vi "(SubVI) Change ADC and DAC Rate of Stage_YCC.vi"(0 "ADC Rate for 20bit (ms)":T2(ring)=enum."3750 Hz", 2 "Tab Control":T1(tab), 3 "DAC rate (ms)":dbl=5.0) -> (5 "Sampling Rate for reading (Hz)":dbl, 6 "DAC rate (Hz)":dbl)   [LabVIEW 2014]
uses:
  Main-Stage-PI/(Global) Current handle and LaserPower_YCC.vi
  MCL-dll-Labview 32-bit/Madlib.dll
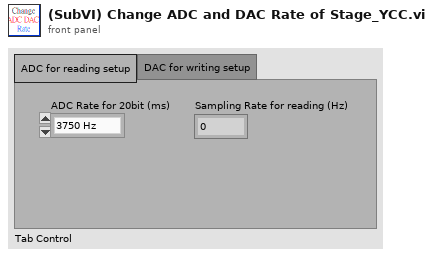
[diagram p1: front panel]
types:
  T1 = enum32{"ADC for reading setup", "DAC for writing setup"}
  T2 = enum16{"50 Hz", "60 Hz", "100 Hz", "500 Hz", "1000 Hz", "2000 Hz", "3750 Hz"}
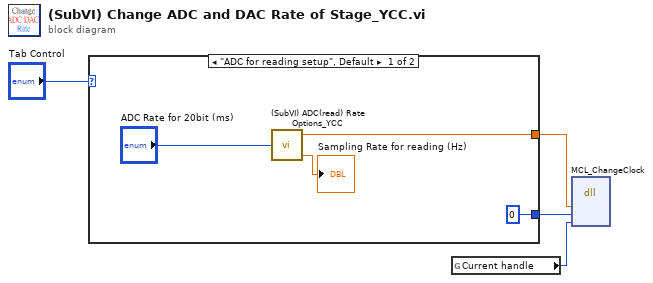
[diagram p0: block diagram]
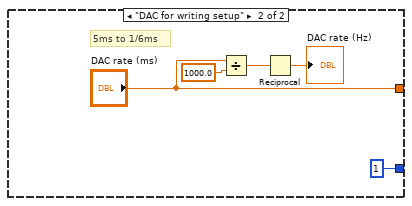
[diagram p2: hidden frame]
diagram:
  n1 = case shown="\"ADC for reading setup\", Default" "Tab Control" {
    tunnel: [0 1] -> w3
    tunnel: [w6 "DAC rate (ms)"] -> w1
    frame "ADC for reading setup", Default {
      n2 = call "(SubVI) ADC(read) Rate Options_YCC.vi"("ADC Rate for 20bit (ms)"="ADC Rate for 20bit (ms)") -> ("Sampling Rate for reading (Hz)"=→"Sampling Rate for reading (Hz)":dbl, "waiting code for Reading (20bits)"=w6:dbl)  [unwired: 3 in]
    }
    frame "DAC for writing setup" {
      # "5ms to 1/6ms"
      n3 = Divide(x="DAC rate (ms)", y=1000.0) -> (x/y=w12:dbl)
      n4 = Reciprocal(x=w12) -> (1/x=→"DAC rate (Hz)":dbl)
    }
  }
  n5 = global read "(Global) Current handle and LaserPower_YCC.vi" "Current handle"() -> (w4:i32)
  n6 = dll-call lib="C:/Users/hwlab/OneDrive - g.ntu.edu.tw/OT/YCC's OT-PI/Main-Stage-Based/SubVI-Stage-Based/MCL-dll-Labview 32-bit/Madlib.dll" fn="MCL_ChangeClock" label="MCL_SingleWriteN"("milliseconds"=w1, "clock"=w3, "handle"=w4) -> ()  [unwired: 7 in, 2 out]
